vi "Test Case - When Constructed - Returns Configured Value.vi"() -> ()   [LabVIEW 2017, in "Test Result.Tests.lvlib"]
uses:
  Test Result.Tests.lvlib
  Test Result/Test Result.lvclass/Test Result.ctl
  Test Result/Get Test Case.vi
  Test Case/Test Case.lvclass
  Test Result/Test Result.lvclass
  <vilib>/PNR/Transparent Assertions/Transparent Assertions/Transparent Assertions.lvlib
panel:
  out "error out":errorcluster
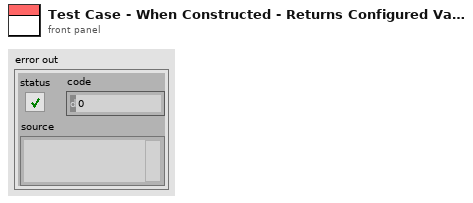
[diagram p1: front panel]
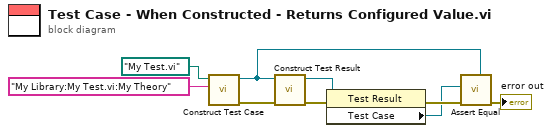
[diagram p0: block diagram]
diagram:
  n1 = call "Construct Test Case.vi"("Qualified Name"="My Library:My Test.vi:My Theory", "Path"=path "My Test.vi") -> ("error out"=w5:errorcluster, "Test Case out"=w4:refnum<class "Test Case.lvclass">)  [unwired: 8 in]
  n2 = call "Construct Test Result.vi"("error in (no error)"=w5, "Test Case"=w4) -> ("error out"=w8:errorcluster, "Test Result"=w9:refnum<class "Test Result.lvclass">)  [unwired: 8 in]
  n3 = property class="Test Result"(reference=w9, error in=w8) -> (error out=w7:errorcluster, "Test Case"=w6:refnum<class "Test Case.lvclass">)  [unwired: 1 out]
  n4 = call <vilib>:"Assert Equal.vi"("Expected"=w4, "error in (no error)"=w7, "Actual"=w6) -> ("error out"=→"error out":errorcluster)  [unwired: 8 in]
